vi "DVR to Refnum.vi"(11 "Data Value Reference in":refnum<data-value>) -> (3 "Refnum out":T1)   [LabVIEW 2019, in "HTTP Client Extensions.lvlib" / "Get Async.lvlib"]
uses:
  Get Async.lvlib
  controls/Refnum Type.ctl
  controls/Refnum Type - Enum.ctl
  HTTP GET Async/GET Async.lvclass
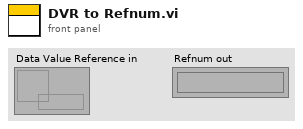
[diagram p1: front panel]
types:
  T1 = typedef "HTTP Client Extensions.lvlib/Get Async.lvlib/Refnum Type.ctl" = refnum<k1>
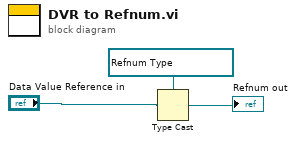
[diagram p0: block diagram]
diagram:
  w1 = T1 refnum items=["HTTP GET Async"] ("get async handle")
  n1 = Type Cast(type=w1, x="Data Value Reference in") -> (*(type *) &x=→"Refnum out":T1)
